vi "Get Owning Ballard ARINC-429 Custom Device.vi"(8 "error in":errorcluster, 11 "item ref in":T1 format="%.0x") -> (0 "error out":errorcluster, 2 "owning Ballard ARINC-429 custom device":T1=18446744073709551615 format="%.0x", 3 "item ref out":T1 format="%.0x")   [LabVIEW 2020, in "Ballard ARINC 429 Scripting.lvlib"]
uses:
  Ballard ARINC 429 Scripting.lvlib
  Constants.vi
  <vilib>/NI VeriStand/Custom Device Tools/Custom Device Utility Library/Custom Device Utility Library.lvlib
  <vilib>/NI VeriStand/Custom Device Tools/Custom Device Utility Library/Search Direction.ctl
  <vilib>/NI VeriStand/Custom Device API/Custom Device Item Ref.ctl
  <vilib>/NI VeriStand/Custom Device API/Custom Device API.lvlib
  <vilib>/NI VeriStand/Custom Device Tools/Custom Device Utility Library/NI VeriStand - Search for Item by GUID.vi
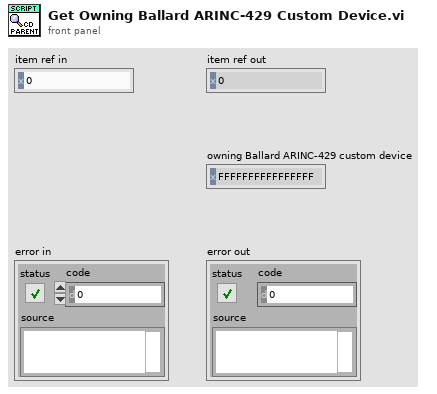
[diagram p1: front panel]
types:
  T1 = typedef "Custom Device API.lvlib/Custom Device Item Ref.ctl" = u64
  T2 = typedef "Custom Device Utility Library.lvlib/Search Direction.ctl" = enum16{"Down", "Up"}
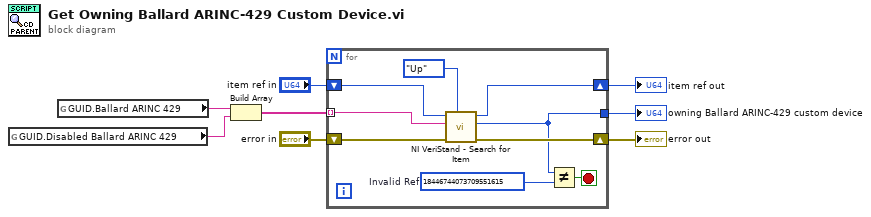
[diagram p0: block diagram]
diagram:
  n1 = global read "Constants.vi" "GUID.Disabled Ballard ARINC 429"() -> (w3:string)
  n2 = global read "Constants.vi" "GUID.Ballard ARINC 429"() -> (w4:string)
  n3 = Build Array(w4, w3) -> (w1:string[])
  n4 = for {
    tunnel: w1 -> [w15] mode=indexing
    shift-right: [w13] -> w5
    shift-left: "item ref in" -> [w17]
    shift-right: [w14] -> w6
    shift-left: "error in" -> [w16]
    tunnel: [w11] -> w2
    stop <- w10 stop-if-true
    w9 = T1 18446744073709551615  # Invalid Ref
    n5 = call-poly <vilib>:"NI VeriStand - Search for Item.vi"("Direction (Down)"=Search_Direction."Up", "error in"=w16, "Item GUID"=w15, "Section Ref in"=w17) -> ("error out"=w14:errorcluster, "Item Ref"=w11:T1, "Section Ref out"=w13:T1)  [unwired: 4 in, 1 out]
    n6 = Not Equal?(x=w11, y=w9) -> (x != y?=w10:bool)
  }
  "owning Ballard ARINC-429 custom device" <- w2
  "error out" <- w6
  "item ref out" <- w5
